vi "GenerateUsers.vi"(8 "error in (no error)":errorcluster) -> (0 "error out":errorcluster)   [LabVIEW 2017]
doc: "Use this template to build a VI to use as a subVI."
uses:
  <vilib>/addons/Database/Connection.llb/DB Tools Open Connec (Path).vi
  <vilib>/addons/Database/_DB Variant To Data/Database Variant To Data.xnode
  <vilib>/addons/Database/NI_Database_API.lvlib
panel:
  out "Active":bool=TRUE
  out "Affiliation":string="Weizmann Institute of Science"
  out "Phone":string="0549303801"
  in  "Active":bool=TRUE
  in  "Affiliation":string="Weizmann Institute of Science"
  in  "Phone":string="0000"
  out "Load Image":T1(plugin-control)
  out "Write Image":T1(plugin-control)
  in  "File Path":path=path "C:/Users/OmerLab/Downloads/Lior Segev.jpg"
  in  "index":i32=5
  in  "Name":string="Lior"
  in  "Surname":string="Segev"
  in  "Password":string="None"
  in  "Title":string="Dr."
  in  "Write Button":bool
  in  "Read Button":bool
  in  "stop 2":bool
  in  "Stop":bool
  out "min temperature value":dbl format="%#.6g"
  out "max temperature value":dbl format="%#.6g"
  out "min pressure value":dbl format="%#.6g"
  out "max pressure value":dbl format="%#.6g"
  out "Core Temperature":dbl[](graph)
  out "Core Pressure":dbl[](graph)
  in  "index (row)":i32=4
  out "data 4":string="Dr."
  out "data 3":string="None"
  out "data 2":string="Segev"
  out "data":string="Lior"
  # "Edit Users Interface"
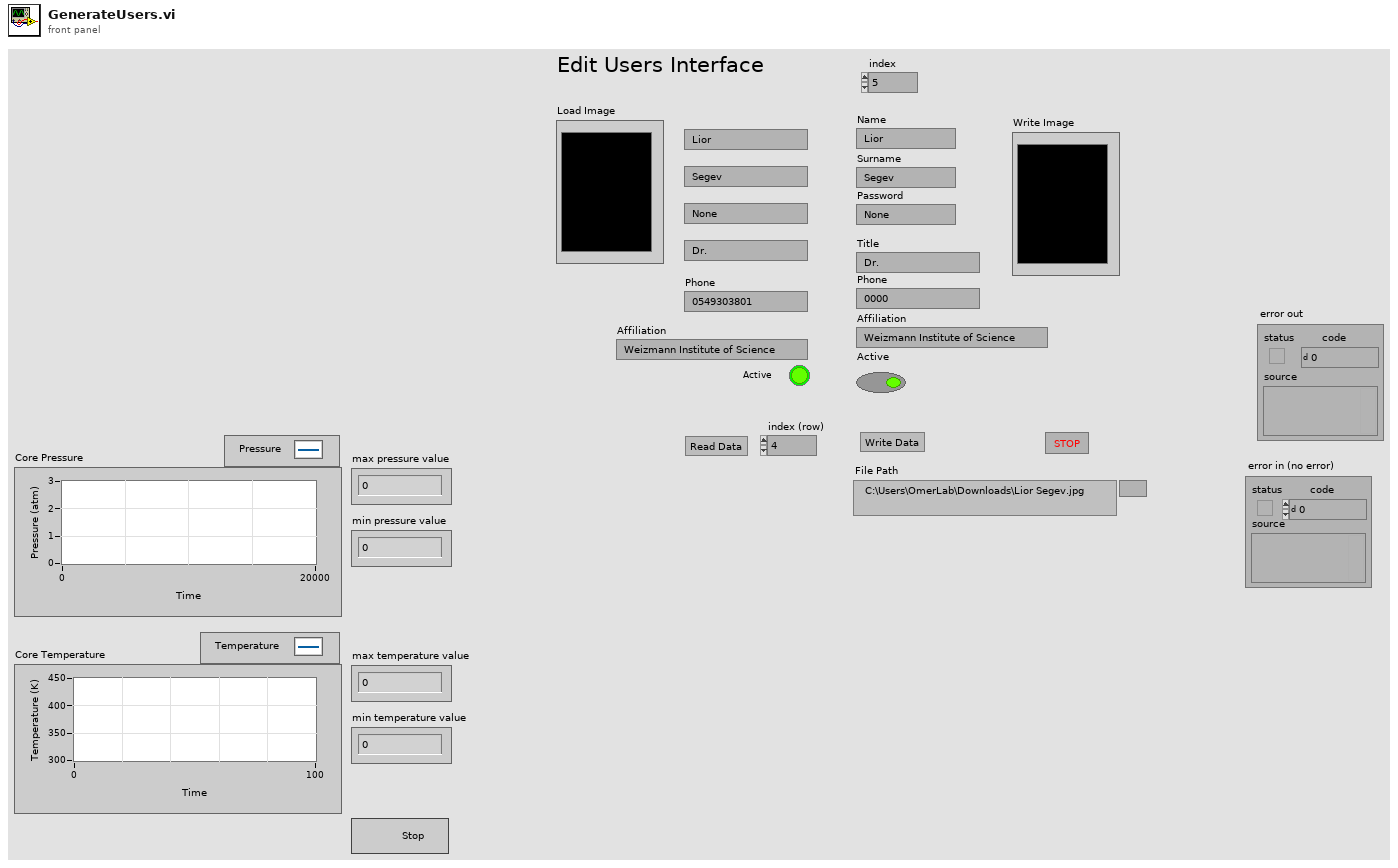
[diagram p1: front panel]
types:
  T1 = typedef "IMAQ Image.ctl" = refnum<image>
  T2 = typedef "NI_Database_API.lvlib/Conn ObjectReference.ctl" = refnum<k1>
  T3 = typedef "Image Type" = u32
  T4 = cluster{"index":i32, "Name":string, "Surname":string, "Password":string, "Title":string, "FileString":string, "Phone":string, "Affiliation":string, i16}
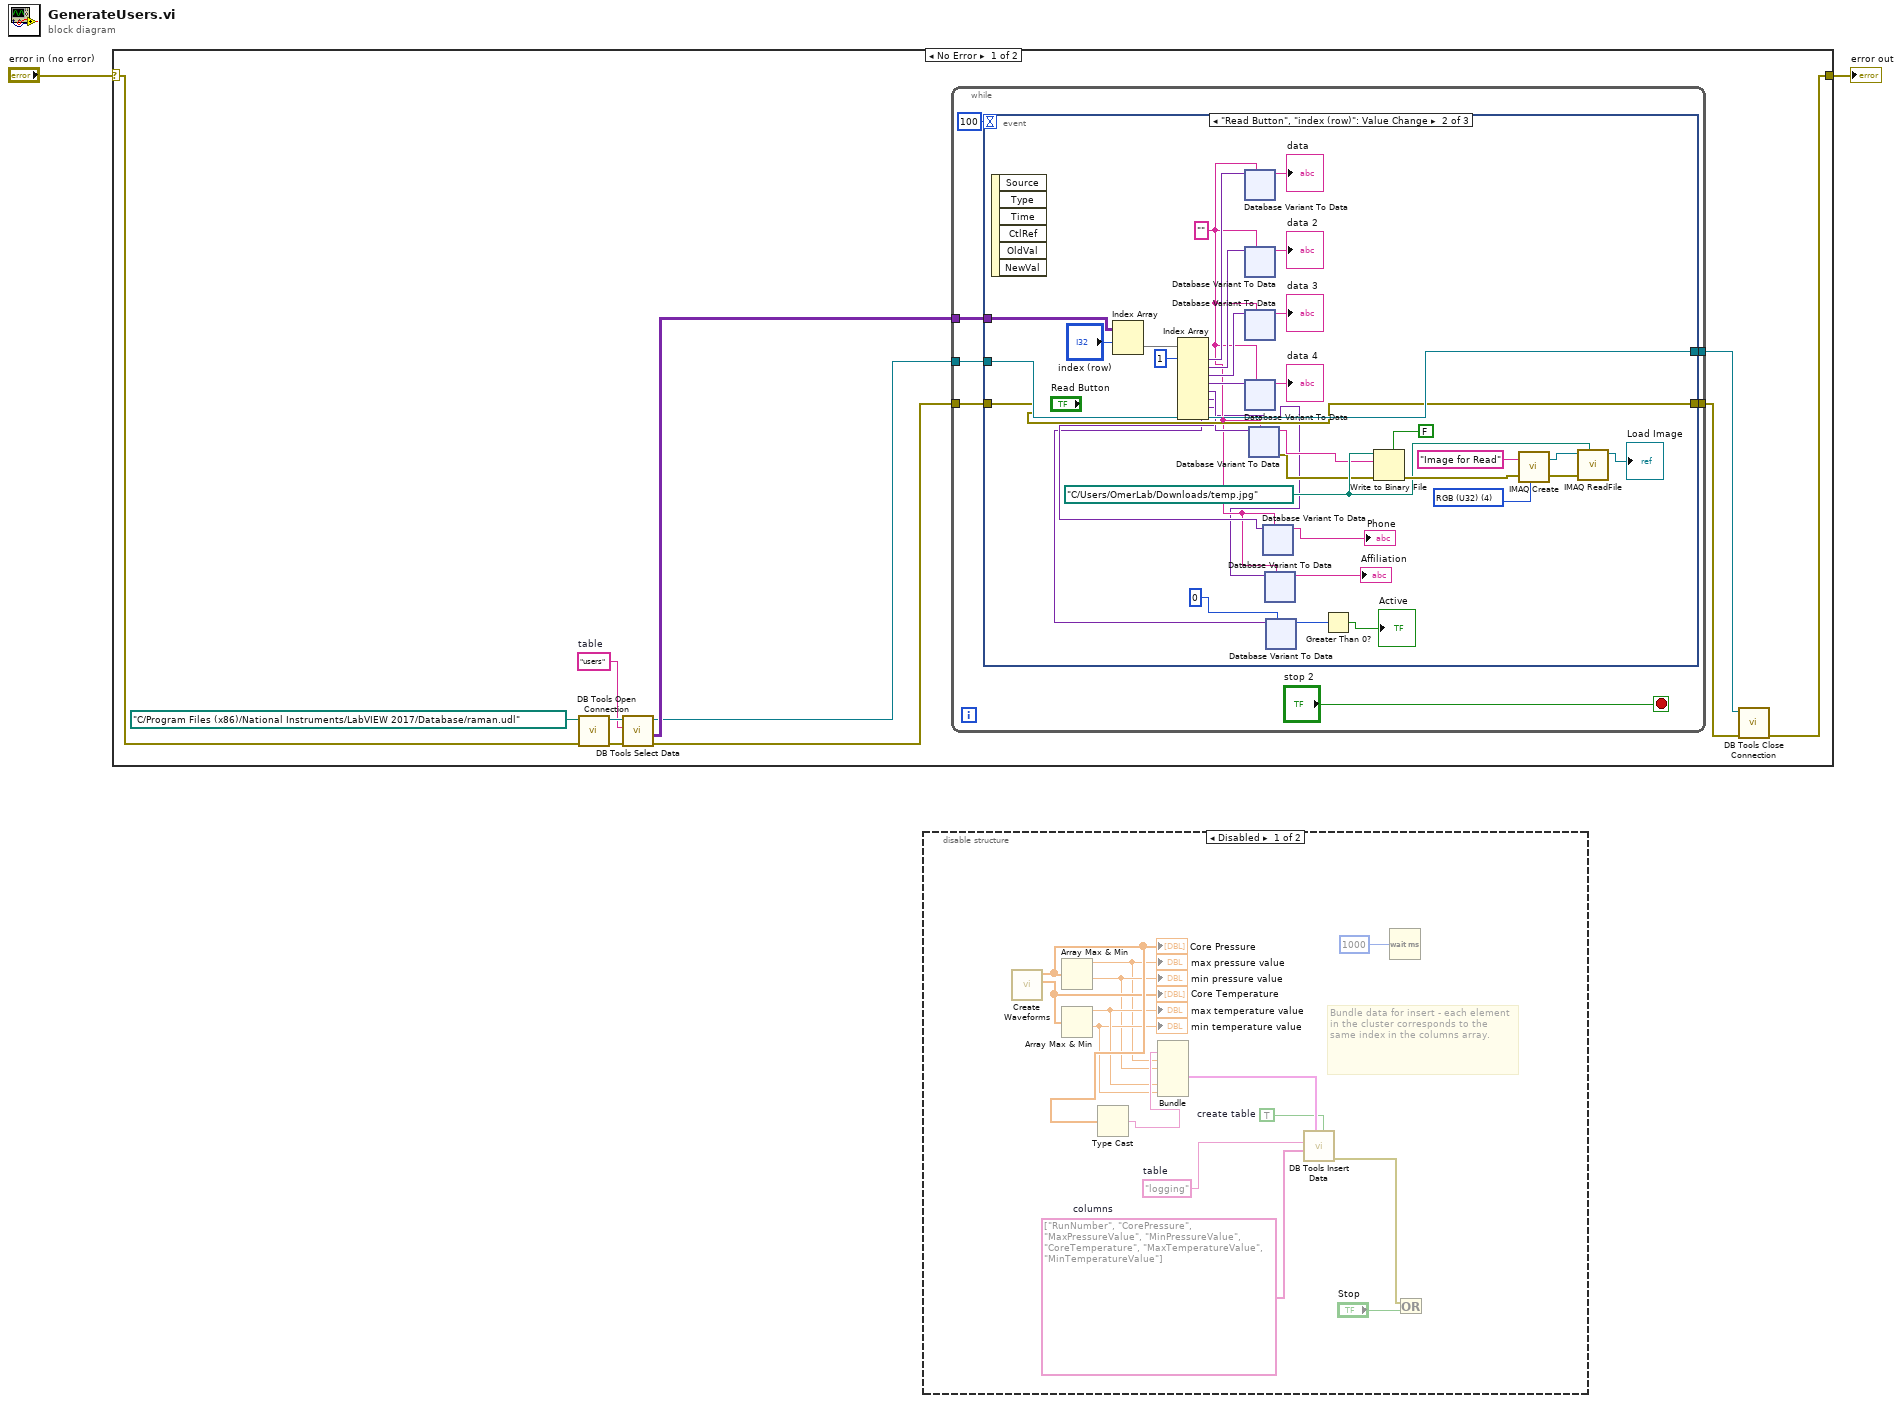
[diagram p0: block diagram]
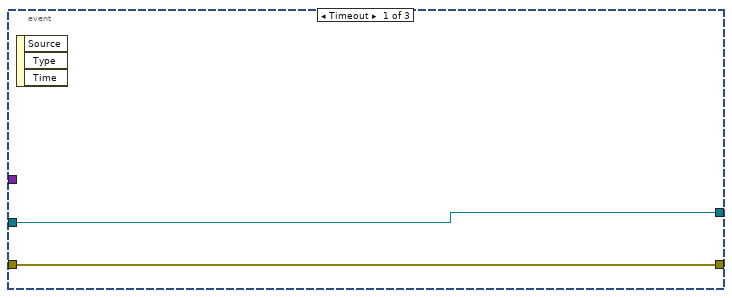
[diagram p3: hidden frame]
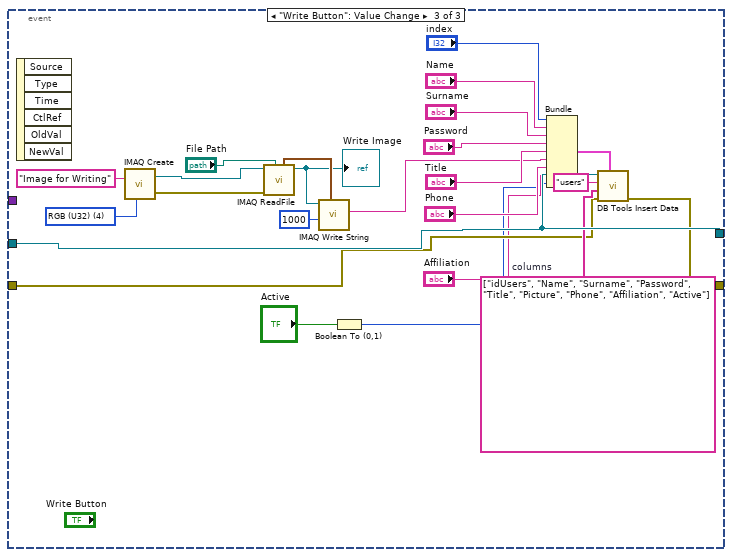
[diagram p4: hidden frame]
diagram:
  n1 = case shown="No Error" "error in (no error)" {
    selector: "error in (no error)" -> [w9 w337]
    tunnel: [w3 w337] -> w1
    frame No Error {
      w11 = "users"  # table
      n2 = call-poly <vilib>:"DB Tools Open Connection.vi"("error in (no error)"=w9, "connection information"=path "C:/Program Files (x86)/National Instruments/LabVIEW 2017/Database/raman.udl") -> ("error out"=w13:errorcluster, "connection reference"=w12:T2)  [unwired: 6 in]
      n3 = call <vilib>:"DB Tools Select Data.vi"("error in (no error)"=w13, "table"=w11, "connection reference"=w12) -> ("error out"=w7:errorcluster, "data"=w8:variant[][], "connection reference out"=w6:T2)  [unwired: 3 in]
      n4 = while {
        tunnel: w8 -> [w18]
        tunnel: w7 -> [w17]
        tunnel: w6 -> [w16]
        tunnel: [w15] -> w5
        tunnel: [w14] -> w4
        stop <- "stop 2" stop-if-true
        n5 = event shown="[1] \"Read Button\", \"index (row)\": Value Change" {
          selector: _ -> [_ _ _]
          dyn-events: _ -> [_ _ _]
          timeout: 100 -> [_ _ _]
          tunnel: w18 -> [_ w45 _]
          tunnel: w17 -> [w21 w43 w327]
          tunnel: w16 -> [w22 w44 w336]
          tunnel: [w21 w43 w326] -> w15
          tunnel: [w22 w44 w336] -> w14
          event Timeout {
            n6 = event-data() -> ()  [unwired: 1 in, 3 out]
          }
          event "Read Button", "index (row)": Value Change {
            w35 = path "C:/Users/OmerLab/Downloads/temp.jpg" ("file (use dialog)")
            w41 = T3 4 items=["Grayscale (U8)", "Grayscale (I16)", "Grayscale (SGL)", "Complex (CSG)", "RGB (U32)", "HSL (U32)", "RGB (U64)", "Grayscale (U16)"] ("Image Type")
            w29 = ""
            n7 = event-data() -> ()  [unwired: 1 in, 6 out]
            n8 = Index Array(array=w45, index (row)="index (row)") -> (element=w47:variant[])  [unwired: 1 in]
            n9 = Index Array(array=w47, index #1=1 ("index")) -> (element #1=w48:variant, element #2=w49:variant, element #3=w50:variant, element #4=w54:variant, element #5=w40:variant, element #6=w31:variant, element #7=w28:variant, element #8=w26:variant)  [unwired: 7 in]
            n10 = xnode "Database Variant To Data"("database variant"=w48, "type"=w29) -> ("data"=→"data":string)  [unwired: 1 in, 1 out]
            n11 = xnode "Database Variant To Data"("database variant"=w49, "type"=w29) -> ("data"=→"data 2":string)  [unwired: 1 in, 1 out]
            n12 = xnode "Database Variant To Data"("database variant"=w50, "type"=w29) -> ("data"=→"data 3":string)  [unwired: 1 in, 1 out]
            n13 = xnode "Database Variant To Data"("database variant"=w54, "type"=w29) -> ("data"=→"data 4":string)  [unwired: 1 in, 1 out]
            n14 = xnode "Database Variant To Data"("database variant"=w40, "type"=w29) -> ("data"=w33:string, "error out"=w32:errorcluster)  [unwired: 1 in]
            n15 = xnode "Database Variant To Data"("database variant"=w31, "type"=w29) -> ("data"=→"Phone":string)  [unwired: 1 in, 1 out]
            n16 = xnode "Database Variant To Data"("database variant"=w28, "type"=w29) -> ("data"=→"Affiliation":string)  [unwired: 1 in, 1 out]
            n17 = xnode "Database Variant To Data"("database variant"=w26, "type"=i16 0 ("0, 1")) -> ("data"=w24:i16)  [unwired: 1 in, 1 out]
            n18 = Greater Than 0?(x=w24) -> (x > 0?=→"Active":bool)
            n19 = Write to Binary File(file (use dialog)=w35, data=w33, error in=w32, 5:FALSE ("prepend array or string size? (T)")) -> (error out=w38:errorcluster)  [unwired: 2 in, 2 out]
            n20 = call "IMAQ Create"("Image Name"="Image for Read", "Image Type"=w41, "error in (no error)"=w38) -> ("New Image"=w36:T1, "error out"=w37:errorcluster)  [unwired: 1 in, 1 out]
            n21 = call "IMAQ ReadFile"("File Path"=w35, "error in (no error)"=w37, "Image"=w36) -> ("Image Out"=→"Load Image":T1)  [unwired: 4 in, 4 out]
          }
          event "Write Button": Value Change {
            w318 = T3 4 items=["Grayscale (U8)", "Grayscale (I16)", "Grayscale (SGL)", "Complex (CSG)", "RGB (U32)", "HSL (U32)", "RGB (U64)", "Grayscale (U16)"] ("Image Type")
            w334 = string[] ["idUsers", "Name", "Surname", "Password", "Title", "Picture", "Phone", "Affiliation", "Active"]  # columns
            n22 = event-data() -> ()  [unwired: 1 in, 6 out]
            n23 = call "IMAQ Create"("Image Name"="Image for Writing", "Image Type"=w318) -> ("New Image"=w323:T1, "error out"=w321:errorcluster)  [unwired: 2 in, 1 out]
            n24 = call "IMAQ ReadFile"("File Path"="File Path", "error in (no error)"=w321, "Image"=w323) -> ("Image Out"=w324:T1, "Color Palette out"=w325:cluster{"Red":u8, "Green":u8, "Blue":u8}[])  [unwired: 4 in, 3 out]
            "Write Image" <- w324
            n25 = call-poly "IMAQ Write String"("Color Palette"=w325, "Image Quality"=u32 1000, "Image"=w324) -> ("FileString"=w317:string)  [unwired: 6 in, 2 out]
            n26 = Boolean To (0,1)(Boolean="Active") -> (0, 1=w313:i16)
            n27 = Bundle("index"="index", "Name"="Name", "Surname"="Surname", "Password"="Password", "Title"="Title", "FileString"=w317, "Phone"="Phone", "Affiliation"="Affiliation", w313) -> (w328:T4)  [unwired: 1 in]
            n28 = call <vilib>:"DB Tools Insert Data.vi"("data"=w328, "error in (no error)"=w327, "columns"=w334, "table"="users", "connection reference"=w336) -> ("error out"=w326:errorcluster)  [unwired: 5 in, 1 out]
          }
        }
      }
      n29 = call <vilib>:"DB Tools Close Connection.vi"("error in (no error)"=w5, "connection reference"=w4) -> ("error out"=w3:errorcluster)  [unwired: 5 in]
    }
    frame Error {
    }
  }
  "error out" <- w1
  n30 = disable-structure shown="Disabled" {
    frame Disabled {
      w340 = string[] ["RunNumber", "CorePressure", "MaxPressureValue", "MinPressureValue", "CoreTemperature", "MaxTemperatureValue", "MinTemperatureValue"]  # columns
      w339 = "logging"  # table
      w341 = TRUE  # create table
      # "Bundle data for insert - each element in the cluster corresponds to the same index in the columns array."
      n31 = call "Create Waveforms.vi"() -> ("core temperature"=w348:dbl[], "core pressure"=w350:dbl[])  [unwired: 10 in]
      "Core Pressure" <- w350
      "Core Temperature" <- w348
      n32 = Array Max & Min(array=w350) -> (max value=w342:dbl, min value=w343:dbl)  [unwired: 2 out]
      "max pressure value" <- w342
      "min pressure value" <- w343
      n33 = Array Max & Min(array=w348) -> (max value=w345:dbl, min value=w344:dbl)  [unwired: 2 out]
      "max temperature value" <- w345
      "min temperature value" <- w344
      n34 = Type Cast(x=w350) -> (*(type *) &x=w351:string)  [unwired: 1 in]
      n35 = Bundle(w351, w342, w343, w345, w344) -> (w346:cluster{void, string, dbl, dbl, void, dbl, dbl})  [unwired: 3 in]
      n36 = call <vilib>:"DB Tools Insert Data.vi"("create table? (F)"=w341, "data"=w346, "columns"=w340, "table"=w339) -> ("error out"=w349:errorcluster)  [unwired: 6 in, 1 out]
      n37 = Wait (ms)(milliseconds to wait=u32 1000) -> ()  [unwired: 1 out]
      n38 = Or(x=w349, y="Stop") -> ()  [unwired: 1 out]
    }
    frame Enabled {
    }
  }
